vi "Measure All (Last).vi"(0 "VISA resource name out":refnum<visa-resource-name>, 11 "error in (no error)":errorcluster) -> (4 "VISA resource name out 2":refnum<visa-resource-name>, 6 "Raw String":string, 8 "Numeric Array":dbl[](array[numeric]), 10 "String Array":string[](array[string]), 15 "error out 2":errorcluster)   [LabVIEW 2013, in "Fluke 2625A.lvlib"]
uses:
  <instrlib>/Fluke 2625A/Fluke 2625A.lvlib
panel:
  out "substring":string
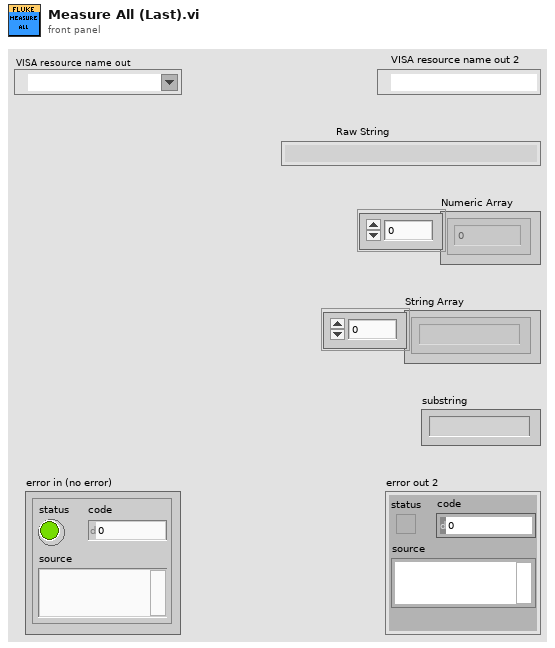
[diagram p1: front panel]
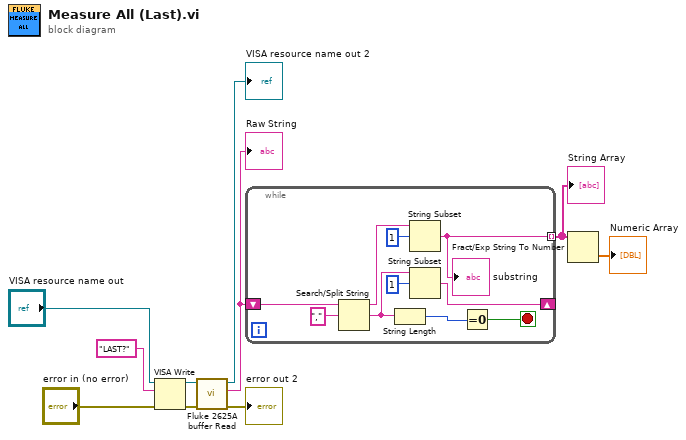
[diagram p0: block diagram]
diagram:
  n1 = VISA Write(VISA resource name="VISA resource name out", write buffer="LAST?", error in (no error)="error in (no error)") -> (VISA resource name out=w8:refnum<visa-resource-name>, error out=w7:errorcluster)  [unwired: 1 out]
  n2 = call <instrlib>:"Fluke 2625A buffer Read.vi"("error out"=w7, "VISA resource name out"=w8) -> ("error out 2"=→"error out 2":errorcluster, "read buffer"=w4:string, "VISA resource name out 2"=→"VISA resource name out 2":refnum<visa-resource-name>)  [unwired: 7 in]
  "Raw String" <- w4
  n3 = while {
    shift-right: [w12] -> _
    shift-left: w4 -> [w15]
    tunnel: [w11] -> w3 mode=indexing
    stop <- w16 stop-if-true
    n4 = Search/Split String(string=w15, search string/char (-)=",") -> (substring before match=w19:string, match + rest of string=w14:string)  [unwired: 1 in, 1 out]
    n5 = String Length(string=w14) -> (length=w17:i32)
    n6 = String Subset(string=w19, offset (0)=1) -> (substring=w11:string)  [unwired: 1 in]
    "substring" <- w11
    n7 = String Subset(string=w14, offset (0)=1) -> (substring=w12:string)  [unwired: 1 in]
    n8 = Equal To 0?(x=w17) -> (x = 0?=w16:bool)
  }
  "String Array" <- w3
  n9 = Fract/Exp String To Number(string=w3) -> (number=→"Numeric Array":dbl[])  [unwired: 3 in, 1 out]
